vi "Configure Serial Output DMA FIFOs.vi"(0 "fpga interface in":refnum<k20>, 5 "serial output channels":string[](array[string]), 7 "llp packets dma fifo depth (elements)":u32=10240000, 11 "error in (no error)":errorcluster) -> (4 "fpga interface out":refnum<k20>, 15 "error out":errorcluster)   [LabVIEW 2023, in "GettingStarted_Gen_148X_Host.lvlib"]
uses:
  GettingStarted_Gen_148X_Host.lvlib
  Types/148x_Gen_FPGA_Reference.ctl
  <vilib>/rvi/interface/common/niFpgaWaitOnOcc.vi
  <vilib>/rvi/interface/nirviMethod/nirviMethod.xnode
  <vilib>/rvi/errors/niLvFpgaMergeErrorWithErrorCode.vi
  <vilib>/FPGAPlugInAG/Dynamic/niLvFpga_ConfigureFifo_Dynamic.vi
  <vilib>/FPGAPlugInAG/Dynamic/niLvFpga_StartFifo_Dynamic.vi
  <instrlib>/FlexRIO/Automotive Vision Utility/v1/Host/Automotive Vision Utility.lvlib
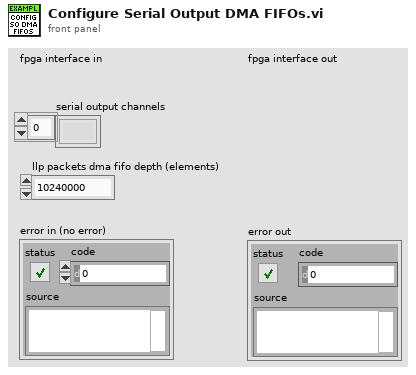
[diagram p1: front panel]
types:
  T1 = typedef "GettingStarted_Gen_148X_Host.lvlib/148x_Gen_FPGA_Reference.ctl" = refnum<k20>
  T2 = typedef "Automotive Vision Utility.lvlib/Serial Channel Type.ctl" = enum16{"Serial Input Channel", "Serial Output Channel", "Unknown Channel Type"}
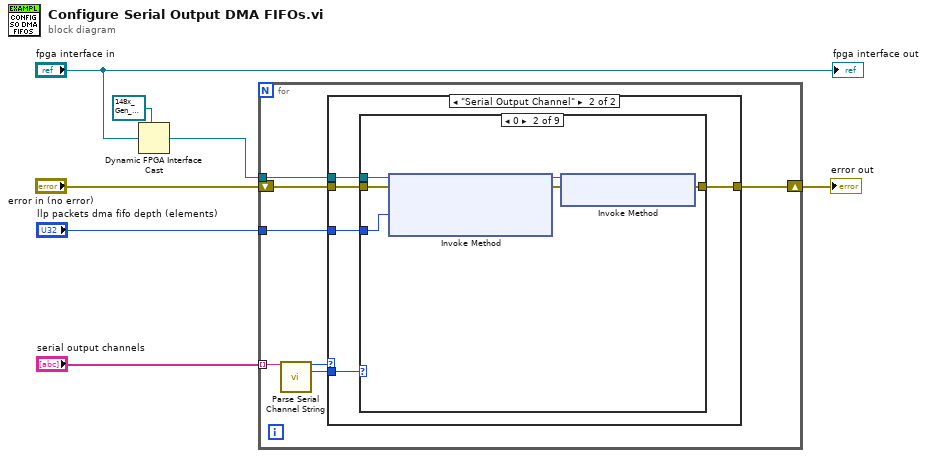
[diagram p0: block diagram]
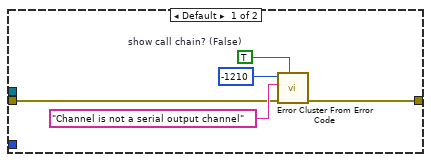
[diagram p2: hidden frame]
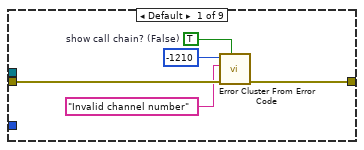
[diagram p3: hidden frame]
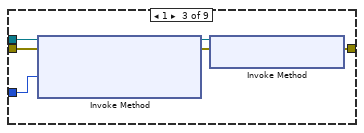
[diagram p4: hidden frame]
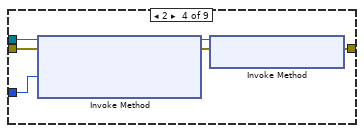
[diagram p5: hidden frame]
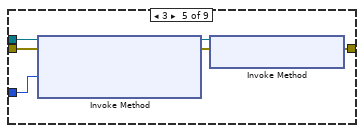
[diagram p6: hidden frame]
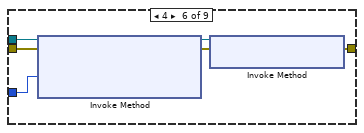
[diagram p7: hidden frame]
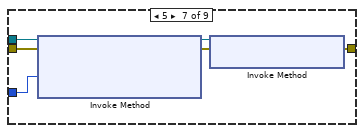
[diagram p8: hidden frame]
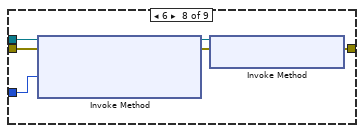
[diagram p9: hidden frame]
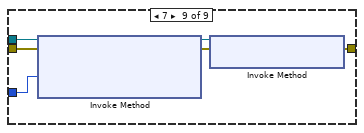
[diagram p10: hidden frame]
diagram:
  n1 = Dynamic FPGA Interface Cast(Session In=T1 refnum ("FPGA VI Reference Out"), Type="fpga interface in") -> (Session Out=w4:T1)
  n2 = for {
    tunnel: "llp packets dma fifo depth (elements)" -> [w13]
    tunnel: w4 -> [w12]
    shift-right: [w11] -> w2
    shift-left: "error in (no error)" -> [w14]
    tunnel: "serial output channels" -> [w10] mode=indexing
    n3 = call <instrlib>:"Parse Serial Channel String.vi"("serial channel string"=w10) -> ("serial channel type"=w9:T2, "channel number"=w8:i32)  [unwired: 13 in]
    n4 = case shown="\"Serial Output Channel\"" w9 {
      tunnel: w14 -> [w16 w24]
      tunnel: w13 -> [_ w23]
      tunnel: w12 -> [_ w22]
      tunnel: [w15 w21] -> w11
      tunnel: w8 -> [_ w20]
      frame Default {
        w17 = TRUE  # show call chain? (False)
        n5 = call <vilib>:"Error Cluster From Error Code.vi"("show call chain? (False)"=w17, "error in (no error)"=w16, "error message (\"\")"="Channel is not a serial output channel" ("error message (\"\")"), "error code (0)"=-1210) -> ("error out"=w15:errorcluster)  [unwired: 5 in]
      }
      frame "Serial Output Channel" {
        n6 = case shown="0" w20 {
          tunnel: w24 -> [w26 w33 w39 w45 w51 w57 w63 w69 w75]
          tunnel: w23 -> [_ w31 w37 w43 w49 w55 w61 w67 w73]
          tunnel: w22 -> [_ w32 w38 w44 w50 w56 w62 w68 w74]
          tunnel: [w27 w30 w36 w42 w48 w54 w60 w66 w72] -> w21
          frame Default {
            w28 = TRUE  # show call chain? (False)
            n7 = call <vilib>:"Error Cluster From Error Code.vi"("show call chain? (False)"=w28, "error in (no error)"=w26, "error message (\"\")"="Invalid channel number" ("error message (\"\")"), "error code (0)"=-1210) -> ("error out"=w27:errorcluster)  [unwired: 5 in]
          }
          frame 0 {
            n8 = xnode "Invoke Method"("FPGA VI Reference In"=w32, "error in"=w33, "Requested Depth"=w31) -> ("FPGA VI Reference Out"=w34:T1, "error out"=w35:errorcluster)  [unwired: 1 out]
            n9 = xnode "Invoke Method"("FPGA VI Reference In"=w34, "error in"=w35) -> ("error out"=w30:errorcluster)  [unwired: 1 out]
          }
          frame 1 {
            n10 = xnode "Invoke Method"("FPGA VI Reference In"=w38, "error in"=w39, "Requested Depth"=w37) -> ("FPGA VI Reference Out"=w40:T1, "error out"=w41:errorcluster)  [unwired: 1 out]
            n11 = xnode "Invoke Method"("FPGA VI Reference In"=w40, "error in"=w41) -> ("error out"=w36:errorcluster)  [unwired: 1 out]
          }
          frame 2 {
            n12 = xnode "Invoke Method"("FPGA VI Reference In"=w44, "error in"=w45, "Requested Depth"=w43) -> ("FPGA VI Reference Out"=w46:T1, "error out"=w47:errorcluster)  [unwired: 1 out]
            n13 = xnode "Invoke Method"("FPGA VI Reference In"=w46, "error in"=w47) -> ("error out"=w42:errorcluster)  [unwired: 1 out]
          }
          frame 3 {
            n14 = xnode "Invoke Method"("FPGA VI Reference In"=w50, "error in"=w51, "Requested Depth"=w49) -> ("FPGA VI Reference Out"=w52:T1, "error out"=w53:errorcluster)  [unwired: 1 out]
            n15 = xnode "Invoke Method"("FPGA VI Reference In"=w52, "error in"=w53) -> ("error out"=w48:errorcluster)  [unwired: 1 out]
          }
          frame 4 {
            n16 = xnode "Invoke Method"("FPGA VI Reference In"=w56, "error in"=w57, "Requested Depth"=w55) -> ("FPGA VI Reference Out"=w58:T1, "error out"=w59:errorcluster)  [unwired: 1 out]
            n17 = xnode "Invoke Method"("FPGA VI Reference In"=w58, "error in"=w59) -> ("error out"=w54:errorcluster)  [unwired: 1 out]
          }
          frame 5 {
            n18 = xnode "Invoke Method"("FPGA VI Reference In"=w62, "error in"=w63, "Requested Depth"=w61) -> ("FPGA VI Reference Out"=w64:T1, "error out"=w65:errorcluster)  [unwired: 1 out]
            n19 = xnode "Invoke Method"("FPGA VI Reference In"=w64, "error in"=w65) -> ("error out"=w60:errorcluster)  [unwired: 1 out]
          }
          frame 6 {
            n20 = xnode "Invoke Method"("FPGA VI Reference In"=w68, "error in"=w69, "Requested Depth"=w67) -> ("FPGA VI Reference Out"=w70:T1, "error out"=w71:errorcluster)  [unwired: 1 out]
            n21 = xnode "Invoke Method"("FPGA VI Reference In"=w70, "error in"=w71) -> ("error out"=w66:errorcluster)  [unwired: 1 out]
          }
          frame 7 {
            n22 = xnode "Invoke Method"("FPGA VI Reference In"=w74, "error in"=w75, "Requested Depth"=w73) -> ("FPGA VI Reference Out"=w76:T1, "error out"=w77:errorcluster)  [unwired: 1 out]
            n23 = xnode "Invoke Method"("FPGA VI Reference In"=w76, "error in"=w77) -> ("error out"=w72:errorcluster)  [unwired: 1 out]
          }
        }
      }
    }
  }
  "error out" <- w2
  "fpga interface out" <- "fpga interface in"
